vi "Colorbar0003.vi"   [LabVIEW 2013]
uses:
  <vilib>/Heliosphere Research LLC/Advanced Plotting Toolkit/api_core/NewPlotType.ctl
  <vilib>/Heliosphere Research LLC/Advanced Plotting Toolkit/Advanced Plotting Toolkit.lvlib
types:
  T1 = typedef "Advanced Plotting Toolkit.lvlib/NewPlotType.ctl" = enum16{"Rectangular Axes", "Polar Axes"}
  T2 = typedef "Advanced Plotting Toolkit.lvlib/PlotID.ctl" = i32
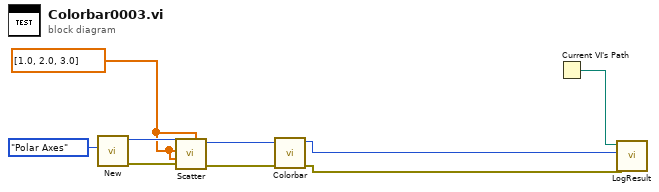
[diagram p0: block diagram]
diagram:
  w2 = dbl[] [1.0, 2.0, 3.0] ("X Data")
  n1 = call <vilib>:"New.vi"("Plot Type"=NewPlotType."Polar Axes") -> ("error out"=w5:errorcluster, "Plot ID"=w6:T2)  [unwired: 9 in]
  n2 = call <vilib>:"Scatter.vi"("Colormap Values"=w2, "error in (no error)"=w5, "Y Data"=w2, "X Data"=w2, "Plot ID"=w6) -> ("error out"=w3:errorcluster, "Plot ID Out"=w4:T2)  [unwired: 5 in]
  n3 = call <vilib>:"Colorbar.vi"("error in (no error)"=w3, "Plot ID"=w4) -> ("error out"=w8:errorcluster, "Plot ID Out"=w7:T2)  [unwired: 8 in]
  n4 = Current VI's Path() -> (path=w9:path)
  n5 = call "LogResult.vi"("Test Result"=w8, "Test Artifact"=w7, "VI Path"=w9) -> ()  [unwired: 9 in]
